vi "helper-build-graph.vi"(6 "Row(2)":i32=2, 9 "Module (OCS)":string="OCS", 10 "filename pattern":string, 11 "lastDays":i8) -> (0 "error out":errorcluster, 2 "size(s)":i32, 3 "Multiple Plots (X Array and Y Array)":cluster{"X":dbl[], "Y":dbl[]})   [LabVIEW 2024]
uses:
  controls/typePathSelector.ctl
  <vilib>/Utility/error.llb/Clear Errors.vi
  <vilib>/Utility/libraryn.llb/Create Directory Recursive.vi
  <vilib>/Utility/file.llb/Read Delimited Spreadsheet (DBL).vi
panel:
  out "filenames":string[](array[string])
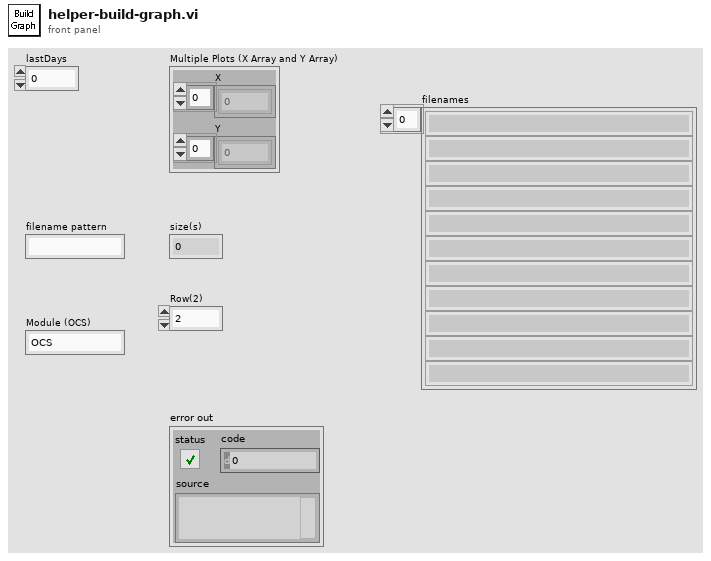
[diagram p1: front panel]
types:
  T1 = typedef "typePathSelector.ctl" = enum16{"DIR_PROCS", "DIR_CONFIG", "DIR_TEMPLATE", "DIR_IO_FILE", "DIR_RECORD", "DIR_LOG", "DIR_RUNTIME", "DIR_PRESET", "DIR_INI"}
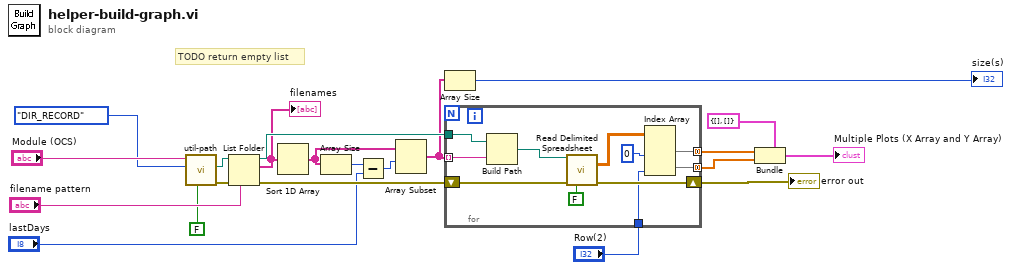
[diagram p0: block diagram]
diagram:
  # "TODO return empty list"
  n1 = call "util-path.vi"("Create Folders?(F)"=FALSE, "Selected Folder (PROCS)"=typePathSelector."DIR_RECORD" ("Enum"), "append path (ie. folder\\filename.*)"="Module (OCS)") -> ("error out"=w21:errorcluster, "SelectedPath"=w12:path)  [unwired: 4 in, 3 out]
  n2 = List Folder(path=w12, pattern="filename pattern", error in=w21) -> (path out=w19:path, filenames=w14:string[], error out=w20:errorcluster)  [unwired: 1 in, 1 out]
  "filenames" <- w14
  n3 = Sort 1D Array(array=w14) -> (sorted array=w18:string[])
  n4 = Array Size(array=w18) -> (size(s)=w15:i32)
  n5 = Subtract(x=w15, y="lastDays") -> (x-y=w17:i32)
  n6 = Array Subset(array=w18, index=w17) -> (w3:string[])  [unwired: 1 in]
  n7 = Array Size(array=w3) -> (size(s)=→"size(s)":i32)
  n8 = for {
    tunnel: [w30] -> w10 mode=concatenating
    tunnel: [w29] -> w11 mode=concatenating
    shift-right: [w31] -> w7
    shift-left: w20 -> [w32]
    tunnel: w19 -> [w25]
    tunnel: w3 -> [w24] mode=indexing
    tunnel: "Row(2)" -> [w22]
    n9 = Build Path(base path=w25, name or relative path=w24) -> (appended path=w23:path)
    n10 = call-poly <vilib>:"Read Delimited Spreadsheet.vi"("file path (dialog if empty)"=w23, "error in (no error)"=w32, "transpose? (F)"=FALSE) -> ("all rows"=w28:dbl[][], "error out"=w31:errorcluster)  [unwired: 7 in, 4 out]
    n11 = Index Array(array=w28, index (col) #1=0 ("disabled index (col)"), index (col) #2=w22) -> (element #1=w29:dbl[], element #2=w30:dbl[])  [unwired: 2 in]
  }
  "error out" <- w7
  n12 = Bundle(cluster=cluster{"X":dbl[], "Y":dbl[]} {"X"=[], "Y"=[]} ("Multiple Plots (X Array and Y Array)"), "X"=w11, "Y"=w10) -> (→"Multiple Plots (X Array and Y Array)":cluster{"X":dbl[], "Y":dbl[]})
